vi "Excel Data Input.vi"(8 "에러 입력":errorcluster caption="에러 입력(에러 없음)", 10 "Name":string, 11 "NI_report 입력":refnum<class "NI_report.lvclass">) -> (0 "에러 출력":errorcluster, 3 "NI_report 출력":refnum<class "NI_report.lvclass">)   [LabVIEW 2020]
uses:
  <vilib>/Utility/NIReport.llb/NI_report.lvclass
  Controls/Cmd_Var Data IO.ctl
  Variables/Global_Cal Info.vi
  Variables/Global_Constant.vi
  <vilib>/Utility/error.llb/Error Cluster From Error Code.vi
  <vilib>/ErrorRing/Error Ring.xnode
  <vilib>/Utility/NIReport.llb/Excel/NI_Excel.lvclass
  <vilib>/addons/_office/NI_ReportGenerationToolkit.lvlib
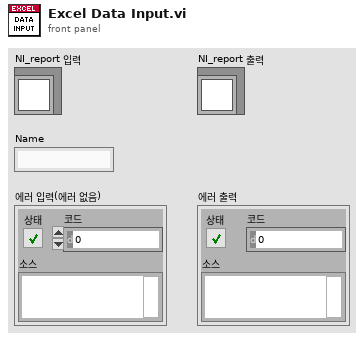
[diagram p1: front panel]
types:
  T1 = typedef "Cmd_Var Data IO.ctl" = enum16{"Condition", "Condition Default", "Condition_Temp", "Resolution", "Resolution Default", "Resolution Old", "Spec", "Spec Default", "Spec Old", "Spec Temp", "Result", "Result2", "Result3", "Result_Temp", "Result_ADJ", "Result_ADJ2", "STD1", "STD2", "STD3", "STD4", "STD5", "STD Temp", "CMC", "CMC Default"}
  T2 = typedef "Clst_Cal Info Global.ctl" = cluster{"등록번호":string, "의뢰기관":string, "기기명":string, "제작회사":string, "형식":string, "기기번호":string, "소분류코드":string, "세부분류코드":string, "교정주기":string, "접수번호":string, "교정일자":string, "교정절차서 1":string, "교정절차서 2":string, "교정절차서 3":string, "접수확인자":string, "인증교정자":string, "기술책임자":string, "KOLAS 유무":string, "진행상태":string, "의뢰기관코드":string, "입고형태":string, "영문성적서?":bool, "합불판정?":bool, "부록?":bool, "절차서번호 1":string, "절차서번호 2":string, "절차서번호 3":string, "교정방식":string, "부서명":string}
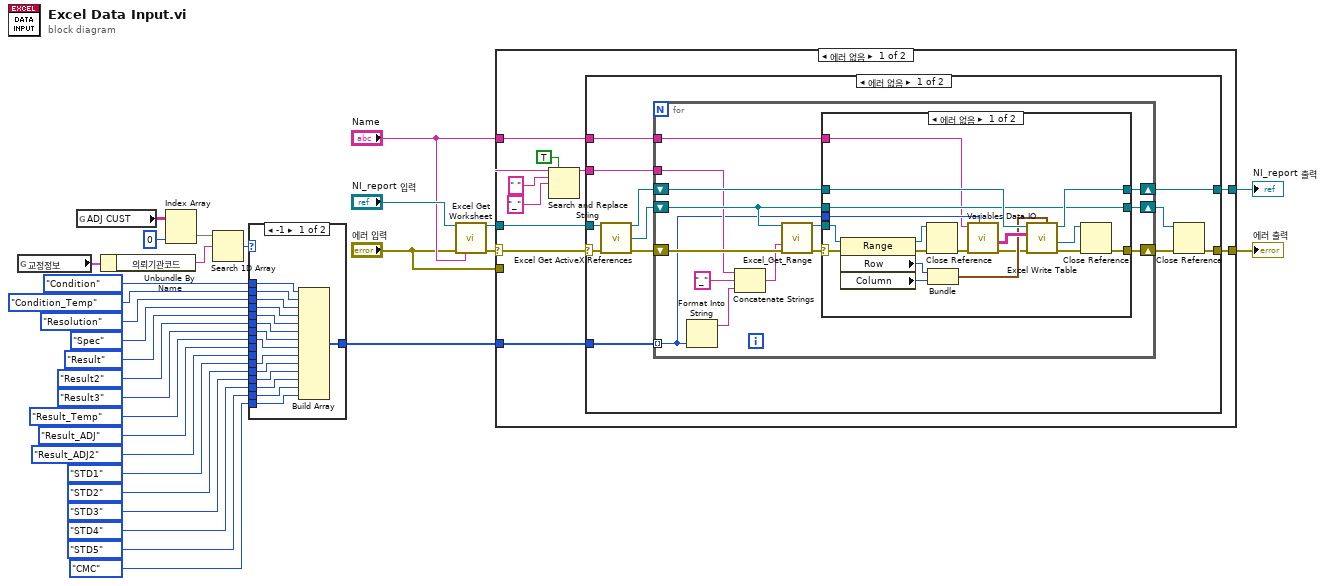
[diagram p0: block diagram]
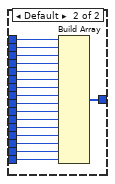
[diagram p2: hidden frame]
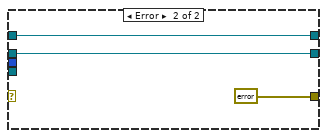
[diagram p3: hidden frame]
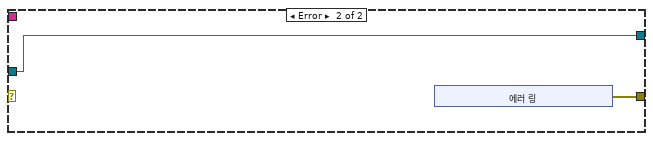
[diagram p4: hidden frame]
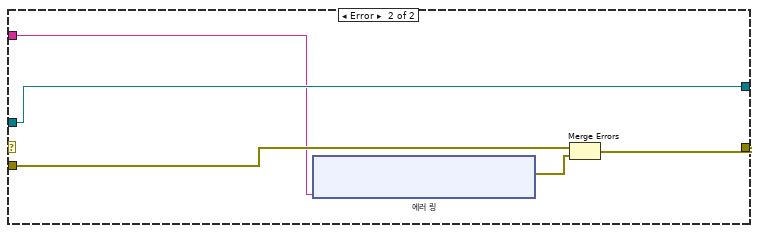
[diagram p5: hidden frame]
diagram:
  n1 = global read "Global_Cal Info.vi" "교정정보"() -> (w2:T2)
  n2 = global read "Global_Constant.vi" "ADJ CUST"() -> (w3:string[][])
  n3 = Unbundle By Name(w2) -> ("의뢰기관코드"=w6:string)
  n4 = Index Array(array=w3, index (col)=0 ("비활성화된 인덱스 (열)")) -> (element=w5:string[])  [unwired: 1 in]
  n5 = Search 1D Array(1D array=w5, element=w6) -> (index of element=w1:i32)  [unwired: 1 in]
  n6 = case shown="-1" w1 {
    tunnel: Cmd_Var_Data_IO."Condition" ("Select") -> [w45 w62]
    tunnel: Cmd_Var_Data_IO."Condition_Temp" ("Select") -> [w44 w61]
    tunnel: Cmd_Var_Data_IO."Resolution" ("Select") -> [w43 w60]
    tunnel: Cmd_Var_Data_IO."Spec" ("Select") -> [w42 w59]
    tunnel: Cmd_Var_Data_IO."Result" ("Select") -> [w41 w58]
    tunnel: Cmd_Var_Data_IO."Result2" ("Select") -> [w40 w57]
    tunnel: Cmd_Var_Data_IO."Result3" ("Select") -> [w39 w56]
    tunnel: Cmd_Var_Data_IO."Result_Temp" ("Select") -> [w38 w55]
    tunnel: Cmd_Var_Data_IO."STD1" ("Select") -> [w37 w54]
    tunnel: Cmd_Var_Data_IO."STD2" ("Select") -> [w36 w53]
    tunnel: Cmd_Var_Data_IO."STD3" ("Select") -> [w35 w52]
    tunnel: Cmd_Var_Data_IO."STD4" ("Select") -> [w34 w51]
    tunnel: Cmd_Var_Data_IO."STD5" ("Select") -> [w33 w50]
    tunnel: Cmd_Var_Data_IO."CMC" ("Select") -> [w32 w49]
    tunnel: [w31 w48] -> w12
    tunnel: Cmd_Var_Data_IO."Result_ADJ" ("Select") -> [_ w47]
    tunnel: Cmd_Var_Data_IO."Result_ADJ2" ("Select") -> [_ w46]
    frame -1 {
      n7 = Build Array(w45, w44, w43, w42, w41, w40, w39, w38, w37, w36, w35, w34, w33, w32) -> (w31:T1[])
    }
    frame Default {
      n8 = Build Array(w62, w61, w60, w59, w58, w57, w56, w55, w47, w46, w54, w53, w52, w51, w50, w49) -> (w48:T1[])
    }
  }
  n9 = call <vilib>:"Excel Get Worksheet.vi"("report in"="NI_report 입력", "error in (no error)"="에러 입력", "name (\"\")"="Name") -> ("report out"=w28:refnum<class "NI_report.lvclass">, "error out"=w10:errorcluster)  [unwired: 11 in]
  n10 = case shown="에러 없음" w10 {
    selector: w10 -> [w63 _]
    tunnel: [w72 w131] -> w30
    tunnel: [w71 w129] -> w29
    tunnel: w28 -> [w70 w131]
    tunnel: w12 -> [w69 _]
    tunnel: "Name" -> [w65 w127]
    tunnel: "에러 입력" -> [_ w128]
    frame No Error {
      n11 = Search and Replace String(replace all?=TRUE ("모두 대체? (거짓)"), input string=w65, search string=" " ("검색 문자열"), replace string="_" ("대체 문자열(\"\")")) -> (result string=w64:string)  [unwired: 4 in, 3 out]
      n12 = case shown="에러 없음" w63 {
        selector: w63 -> [w77 _]
        tunnel: [w84 w121] -> w72
        tunnel: [w74 w120] -> w71
        tunnel: w65 -> [w82 _]
        tunnel: w70 -> [w79 w121]
        tunnel: w69 -> [w78 _]
        tunnel: w64 -> [w73 _]
        frame No Error {
          n13 = call <vilib>:"Excel Get ActiveX References.vi"("report in"=w79, "error in (no error)"=w77) -> ("report out"=w83:refnum<class "NI_report.lvclass">, "Excel._Worksheet"=w81:refnum<k7>, "error out"=w80:errorcluster)  [unwired: 7 in, 4 out]
          n14 = for {
            tunnel: w82 -> [w95]
            tunnel: w78 -> [w90] mode=indexing
            shift-right: [w98] -> w84
            shift-left: w83 -> [w97]
            shift-right: [w96] -> w76
            shift-left: w80 -> [w94]
            shift-right: [w93] -> w75
            shift-left: w81 -> [w92]
            tunnel: w73 -> [w91]
            n15 = Format Into String(w90) -> (resulting string=w86:string)  [unwired: 3 in, 1 out]
            n16 = Concatenate Strings(w91, "_" ("문자열"), w86) -> (w88:string)
            n17 = call <vilib>:"Excel_Get_Range.vi"("Excel._Worksheet"=w92, "name"=w88, "error in (no error)"=w94) -> ("Range"=w89:refnum<k7>, "error out"=w85:errorcluster)  [unwired: 3 in, 8 out]
            n18 = case shown="에러 없음" w85 {
              selector: w85 -> [w104 _]
              tunnel: [w116 w119] -> w98
              tunnel: w97 -> [w115 w119]
              tunnel: [w101 errorcluster {"status"=FALSE, "code"=0, "source"=""} ("error out")] -> w96
              tunnel: w95 -> [w99 _]
              tunnel: w89 -> [w109 _]
              tunnel: w90 -> [w108 _]
              tunnel: [w100 w117] -> w93
              tunnel: w92 -> [w100 w117]
              frame No Error {
                n19 = property class="Range"(reference=w109, error in=w104) -> (reference out=w105:refnum<k7>, error out=w107:errorcluster, "Row"=w110:i32, "Column"=w111:i32)
                n20 = Close Reference(reference=w105, error in (no error)=w107) -> (error out=w106:errorcluster)
                n21 = Bundle("Row"=w110, "Column"=w111) -> (w113:cluster{"Row":i32, "Column":i32})  [unwired: 1 in]
                n22 = call "Variables Data IO.vi"("Select"=w108, "error in"=w106, "Func_ext"=w99) -> ("error out"=w112:errorcluster, "Data Out"=w114:string[][])  [unwired: 6 in, 1 out]
                n23 = call "Excel Write Table.vi"("Address"=w113, "error in"=w112, "table"=w114, "report in"=w115) -> ("error out"=w103:errorcluster, "Range out"=w102:refnum<k7>, "report out"=w116:refnum<class "NI_report.lvclass">)  [unwired: 4 in, 1 out]
                n24 = Close Reference(reference=w102, error in (no error)=w103) -> (error out=w101:errorcluster)
              }
              frame Error {
              }
            }
          }
          n25 = Close Reference(reference=w75, error in (no error)=w76) -> (error out=w74:errorcluster)
        }
        frame Error {
          n26 = xnode "에러 링"() -> ("에러 출력"=w120:errorcluster)
        }
      }
    }
    frame Error {
      n27 = xnode "에러 링"("파라미터 0"=w127) -> ("에러 출력"=w130:errorcluster)
      n28 = Merge Errors(w128, w130) -> (w129:errorcluster)
    }
  }
  "NI_report 출력" <- w30
  "에러 출력" <- w29
